vi "Alarm Lookup (SubVI).vi"(11 "Alarm Code":u16) -> (3 "Alarm Meaning":string)   [LabVIEW 2013]
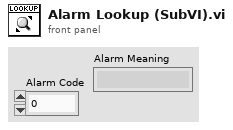
[diagram p1: front panel]
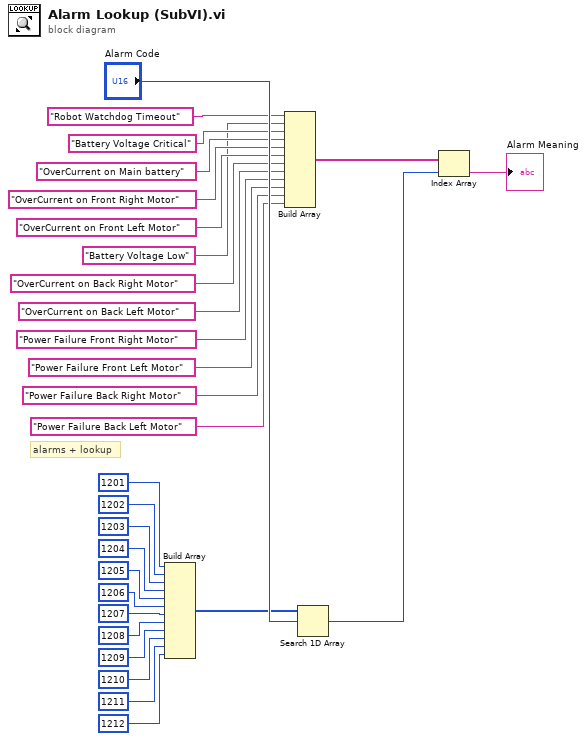
[diagram p0: block diagram]
diagram:
  # "alarms + lookup"
  n1 = Build Array(1201 ("element"), 1202 ("element"), 1203 ("element"), 1204 ("element"), 1205 ("element"), 1206 ("element"), 1207 ("element"), 1208 ("element"), 1209 ("element"), 1210 ("element"), 1211 ("element"), 1212 ("element")) -> (w25:i32[])
  n2 = Build Array("Robot Watchdog Timeout", "Battery Voltage Low", "Battery Voltage Critical", "OverCurrent on Main battery", "OverCurrent on Front Right Motor", "OverCurrent on Front Left Motor", "OverCurrent on Back Right Motor", "OverCurrent on Back Left Motor", "Power Failure Front Right Motor", "Power Failure Front Left Motor", "Power Failure Back Right Motor", "Power Failure Back Left Motor") -> (w27:string[])
  n3 = Search 1D Array(1D array=w25, element="Alarm Code") -> (index of element=w28:i32)  [unwired: 1 in]
  n4 = Index Array(array=w27, index=w28) -> (element=→"Alarm Meaning":string)
